vi "Apply Selected Labels to Control.vi"(8 "error in (no error)":errorcluster, 10 "Alternate Text Select (0)":i32, 11 "Boolean in":refnum<class "Boolean.lvclass">) -> (0 "error out":errorcluster, 3 "Boolean out":refnum<class "Boolean.lvclass">)   [LabVIEW 2017, in "Localization.lvlib" / "Boolean.lvclass"]
doc: "Use the information in the class to apply the selected alternate text from the Additional Labels to the control.\n\nChoose Movement Consulting, LLC"
uses:
  Boolean.lvclass
  C:/Apps/CMC/OpenSource/Localization/Control Info/Control Info.lvclass
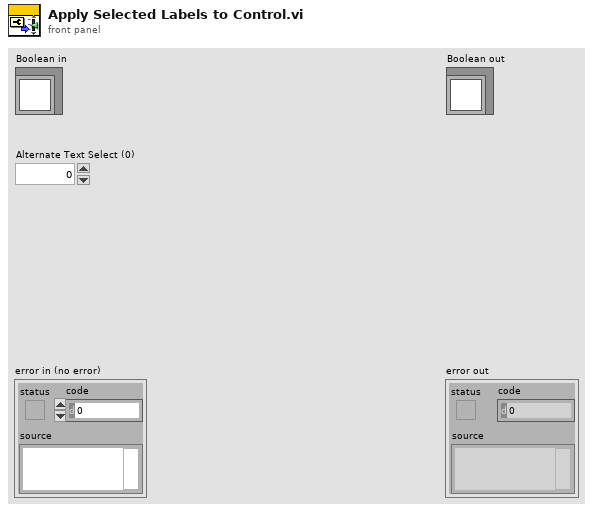
[diagram p1: front panel]
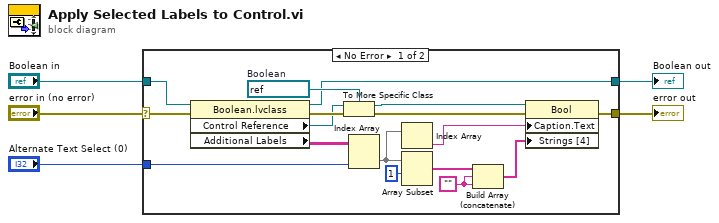
[diagram p0: block diagram]
diagram:
  n1 = case shown="No Error" "error in (no error)" {
    selector: "error in (no error)" -> [w17 w24]
    tunnel: "Boolean in" -> [w16 w23]
    tunnel: [w7 w24] -> w3
    tunnel: [w6 w23] -> w2
    tunnel: "Alternate Text Select (0)" -> [w14 _]
    frame No Error {
      w9 = ""
      w22 = refnum<vi> refnum  # Boolean
      n2 = property class="Boolean.lvclass"(reference=w16, error in=w17) -> (reference out=w6:refnum<class "Boolean.lvclass">, error out=w19:errorcluster, "Control Reference"=w18:refnum<vi>, "Additional Labels"=w15:string[][])
      n3 = To More Specific Class(target class=w22, reference=w18, error in=w19) -> (specific class reference=w21:refnum<vi>, error out=w20:errorcluster)
      n4 = Index Array(array=w15, index (col)=w14) -> (element=w12:string[])  [unwired: 1 in]
      n5 = Index Array(array=w12) -> (element=w13:string)  [unwired: 1 in]
      n6 = Array Subset(array=w12, index=1) -> (w10:string[])  [unwired: 1 in]
      n7 = Build Array (concatenate)(w10, w9, w9) -> (w8:string[])
      n8 = property class="Bool"(reference=w21, error in=w20, "Caption.Text"=w13, "Strings [4]"=w8) -> (error out=w7:errorcluster)  [unwired: 1 out]
    }
    frame Error {
    }
  }
  "error out" <- w3
  "Boolean out" <- w2
